vi "test - Get Assert Event Ref - 2.vi"(8 "error in (no error)":errorcluster, 11 "TestCase in":refnum<class "Get Assert Event Reference tests.lvclass">) -> (0 "error out":errorcluster, 3 "TestCase out":refnum<class "Get Assert Event Reference tests.lvclass">)   [LabVIEW 2016, in "Assert API Components.lvlib" / "Get Assert Event Reference tests.lvclass"]
uses:
  Get Assert Event Reference tests.lvclass
  <vilib>/addons/_JKI Toolkits/VI Tester/TestCase.llb/TestCase.lvclass
  Core/Assert API Components/Assert API Components.lvlib
  C:/Program Files (x86)/National Instruments/LabVIEW 2016/vi.lib/addons/_JKI Toolkits/VI Tester/TestCase.llb/TestCase.lvclass
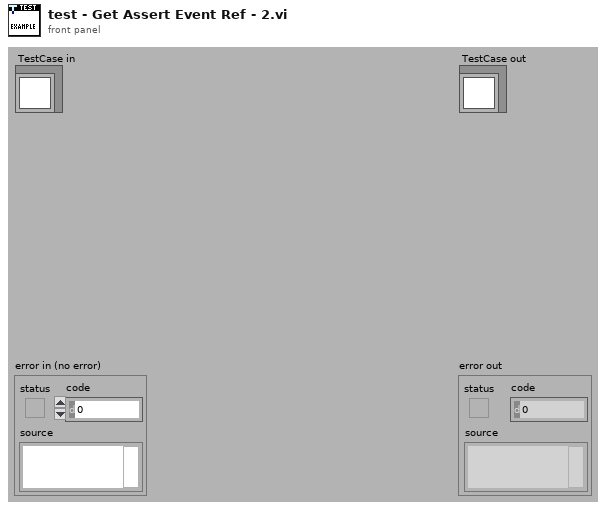
[diagram p1: front panel]
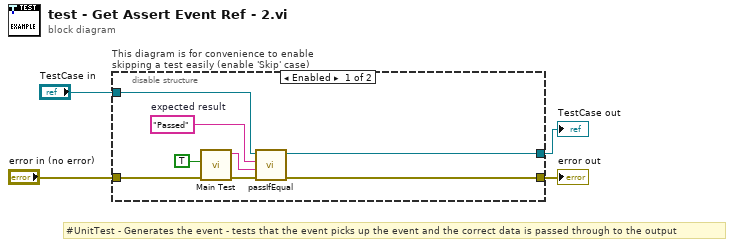
[diagram p0: block diagram]
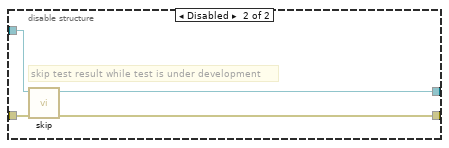
[diagram p2: hidden frame]
diagram:
  # "#UnitTest - Generates the event - tests that the event picks up the event and the correct data is passed through to the output"
  n1 = disable-structure "This diagram is for convenience to enable skipping a test easily (enable 'Skip' case)" shown="Enabled" {
    disable-tunnel: "TestCase in" -> [w11 w16]
    disable-tunnel: [w10 w14] -> w1
    disable-tunnel: [w9 w15] -> w3
    disable-tunnel: "error in (no error)" -> [w5 w13]
    frame Enabled {
      w12 = "Passed"  # expected result
      n2 = call "Main Test.vi"("error in (no error)"=w5, "Generate Event?"=TRUE) -> ("error out"=w6:errorcluster, "Assert Message"=w7:string)  [unwired: 8 in]
      n3 = call-dynamic "passIfEqual.vi"("error in (no error)"=w6, "y"=w7, "x"=w12, "TestCase in"=w11) -> ("error out"=w9:errorcluster, "TestCase out"=w10:refnum<class "Get Assert Event Reference tests.lvclass">)  [unwired: 6 in]
    }
    frame Disabled {
      # "skip test result while test is under development"
      n4 = call <vilib>:"skip.vi"("error in (no error)"=w13, "TestCase in"=w16) -> ("error out"=w15:errorcluster, "TestCase out"=w14:refnum<class "Get Assert Event Reference tests.lvclass">)  [unwired: 8 in]
    }
  }
  "error out" <- w3
  "TestCase out" <- w1
